vi "Phasor Check Backup Calibration Frequency.vi"(9 "Calibration Map Phasor Frequency":dbl[unit], 11 "Calibration Phasor":T1) -> (1 "Same Frequency":bool, 3 "Single Calibration Phasor":cdb)   [LabVIEW 2021, in "Phasor.lvlib"]
uses:
  Calibration Phasor (m, phi).ctl
  4d258da1-ace2-4bae-b161-614013df86fe.vi
  4d258da1-ace2-4bae-b161-614013df86fe.vi/8a80743f-1319-44c8-96b0-3ef8fc688731.vi
  4d258da1-ace2-4bae-b161-614013df86fe.vi/931f4f8f-d8c6-4056-833f-5c8fe97b24b9.vi
  Phasor.lvlib
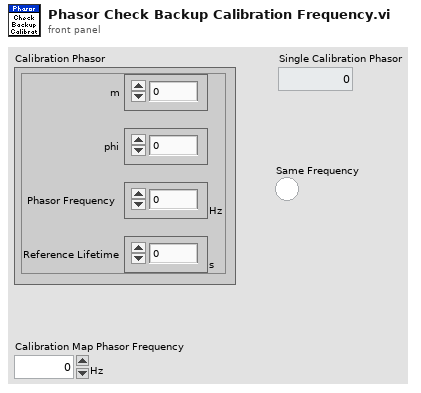
[diagram p1: front panel]
types:
  T1 = typedef "Phasor.lvlib/Calibration Phasor (m, phi).ctl" = cluster{"m":dbl, "phi":dbl, "Phasor Frequency":dbl[unit], "Reference Lifetime":dbl[unit]}
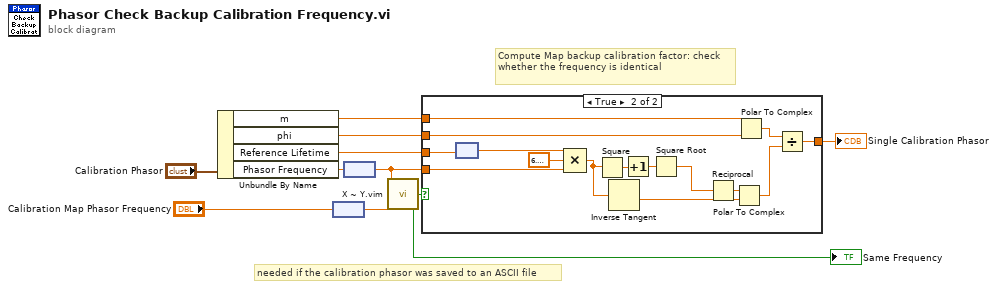
[diagram p0: block diagram]
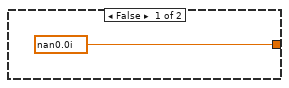
[diagram p2: hidden frame]
diagram:
  # "needed if the calibration phasor was saved to an ASCII file"
  # "Compute Map backup calibration factor: check whether the frequency is identical"
  n1 = Unbundle By Name("Calibration Phasor") -> ("m"=w6:dbl, "phi"=w5:dbl, "Reference Lifetime"=w7:dbl[unit], "Phasor Frequency"=w4:dbl[unit])
  n2 = node("Calibration Map Phasor Frequency") -> (w1:dbl)
  n3 = node(w4) -> (w2:dbl)
  n4 = call "X ~ Y.vim"("X"=w2, "Y"=w1) -> ("X ~= Y?"=w8:bool)  [unwired: 13 in]
  "Same Frequency" <- w8
  n5 = case shown="True" w8 {
    tunnel: [cdb nan+0.0i w13] -> w10
    tunnel: w2 -> [_ w16]
    tunnel: w7 -> [_ w15]
    tunnel: w6 -> [_ w25]
    tunnel: w5 -> [_ w24]
    frame False {
    }
    frame True {
      n6 = node(w15) -> (w14:dbl)
      n7 = Compound Arithmetic op=MULTIPLY(w14, 6.283185307179586, w16) -> (w18:dbl)
      n8 = Square(x=w18) -> (x^2=w19:dbl)
      n9 = Inverse Tangent(1:w18) -> (0:w21:dbl)
      n10 = Increment(x=w19) -> (x+1=w20:dbl)
      n11 = Square Root(x=w20) -> (sqrt(x)=w22:dbl)
      n12 = Reciprocal(x=w22) -> (1/x=w23:dbl)
      n13 = Polar To Complex(1:w21, 2:w23) -> (0:w12:cdb)
      n14 = Polar To Complex(1:w24, 2:w25) -> (0:w26:cdb)
      n15 = Divide(x=w26, y=w12) -> (x/y=w13:cdb)
    }
  }
  "Single Calibration Phasor" <- w10
